vi "TSV_2_LV.vi"(8 "error in (no error)":errorcluster, 11 "file path (dialog if empty)":path) -> (0 "error out":errorcluster)   [LabVIEW 2016, in "VCL_2_DSC.lvclass"]
uses:
  VCL_2_DSC.lvclass
  <vilib>/Utility/file.llb/Read Delimited Spreadsheet (string).vi
  <vilib>/Utility/file.llb/Read Delimited Spreadsheet (DBL).vi
panel:
  out "XY Graph":cluster{timestamp[], dbl[]}(graph)
  out "Value Array":dbl[](array[numeric])
  out "Time Array":timestamp[](array[timestamp])
  out "Name":string
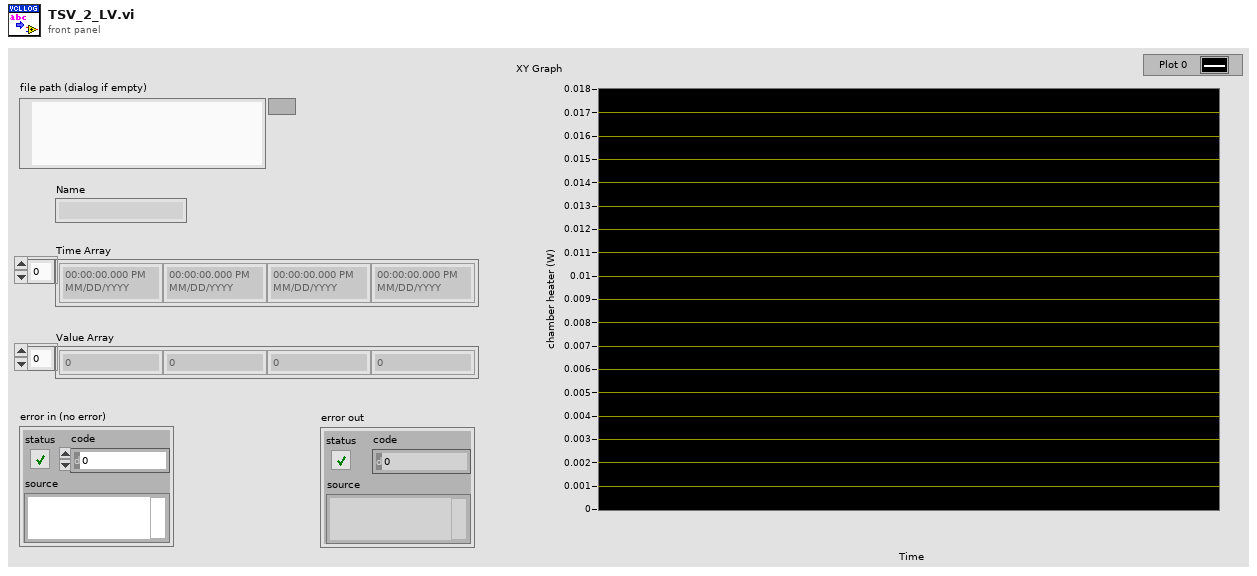
[diagram p1: front panel]
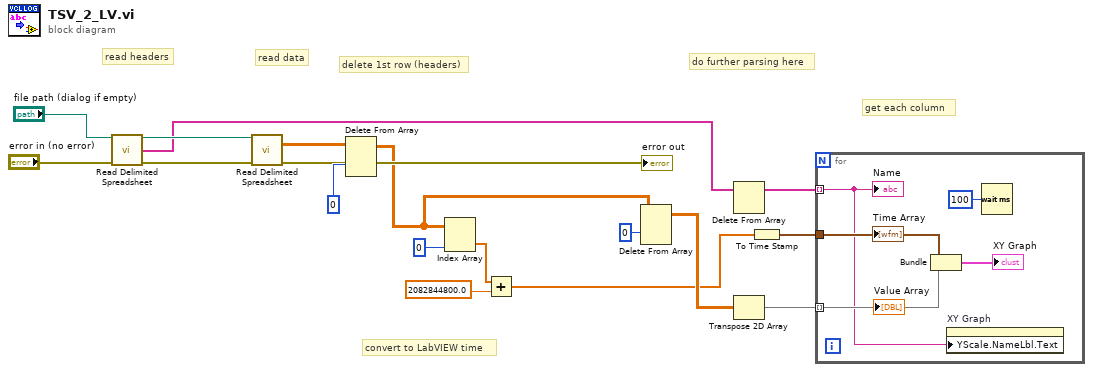
[diagram p0: block diagram]
diagram:
  # "read data"
  # "get each column"
  # "do further parsing here"
  # "convert to LabVIEW time"
  # "delete 1st row (headers)"
  # "read headers"
  n1 = call-poly <vilib>:"Read Delimited Spreadsheet.vi"("file path (dialog if empty)"="file path (dialog if empty)", "error in (no error)"="error in (no error)") -> ("new file path (Not A Path if cancelled)"=w17:path, "first row"=w1:string[], "error out"=w14:errorcluster)  [unwired: 8 in, 3 out]
  n2 = call-poly <vilib>:"Read Delimited Spreadsheet.vi"("file path (dialog if empty)"=w17, "error in (no error)"=w14) -> ("all rows"=w15:dbl[][], "error out"=→"error out":errorcluster)  [unwired: 8 in, 4 out]
  n3 = Delete From Array(array=w15, index (row)=0) -> (array with subset deleted=w2:dbl[][])  [unwired: 2 in, 1 out]
  n4 = Index Array(array=w2, index (col)=0 ("disabled index (col)")) -> (element=w12:dbl[])  [unwired: 1 in]
  n5 = Add(x=w12, y=2082844800.0 ("Numeric 2")) -> (x+y=w3:dbl[])
  n6 = Delete From Array(array=w2, index (row)=0) -> (array with subset deleted=w7:dbl[][])  [unwired: 2 in, 1 out]
  n7 = Delete From Array(array=w1) -> (array with subset deleted=w4:string[])  [unwired: 2 in, 1 out]
  n8 = Transpose 2D Array(2D array=w7) -> (transposed array=w6:dbl[][])
  n9 = To Time Stamp(1:w3) -> (0:w5:timestamp[])
  n10 = for {
    tunnel: w6 -> [w21] mode=indexing
    tunnel: w5 -> [w22]
    tunnel: w4 -> [w19] mode=indexing
    n11 = Bundle(w22, w21) -> (→"XY Graph":cluster{timestamp[], dbl[]})  [unwired: 1 in]
    n12 = property on="XY Graph" class="XYGraph (strict)"("YScale.NameLbl.Text"=w19) -> ()  [unwired: 2 in, 2 out]
    n13 = Wait (ms)(milliseconds to wait=u32 100) -> ()  [unwired: 1 out]
    "Name" <- w19
    "Time Array" <- w22
    "Value Array" <- w21
  }
